vi "Set CPU Pools.vi"(8 "error in (no error)":errorcluster) -> (0 "error out":errorcluster, 2 "Processor Assignment":i32)   [LabVIEW 2014]
uses:
  <vilib>/Utility/RT CPU pool selections.ctl
  <vilib>/NI_Real-Time Target Support.lvlib
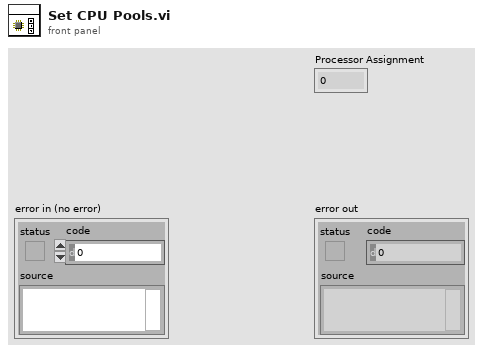
[diagram p1: front panel]
types:
  T1 = typedef "NI_Real-Time Target Support.lvlib/RT CPU pool selections.ctl" = enum16{"System & Timed Structures", "System", "Timed Structures", "Reserved"}
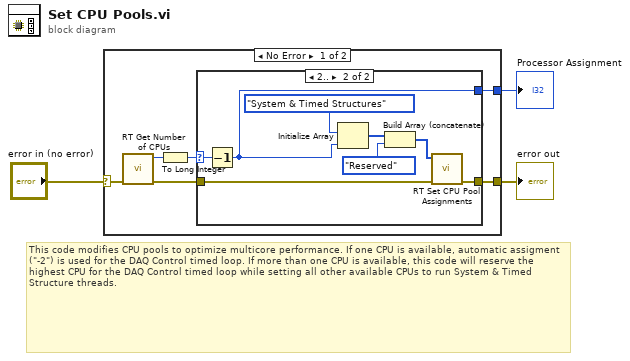
[diagram p0: block diagram]
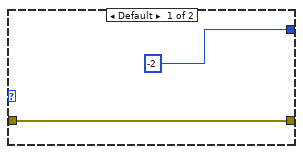
[diagram p2: hidden frame]
diagram:
  # "This code modifies CPU pools to optimize multicore performance. If one CPU is available, automatic assigment (\"-2\") is used for the DAQ Control timed loop. If more than one CPU is available, this code will reserve the highest CPU for the DAQ Control timed loop while setting all other available CPUs to run System & Timed Structure threads."
  n1 = case shown="No Error" "error in (no error)" {
    selector: "error in (no error)" -> [w7 w20]
    tunnel: [w8 w20] -> w3
    tunnel: [w5 _] -> w1
    frame No Error {
      n2 = call <vilib>:"RT Get Number of CPUs.vi"("error in (no error)"=w7) -> ("error out"=w9:errorcluster, "# of CPUs"=w6:u32)  [unwired: 9 in]
      n3 = To Long Integer(number=w6) -> (32bit integer=w4:i32)
      n4 = case shown="2.." w4 {
        selector: w4 -> [_ w13]
        tunnel: w9 -> [w11 w19]
        tunnel: [w11 w18] -> w8
        tunnel: [-2 ("# of CPUs") w12] -> w5
        frame Default {
        }
        frame 2.. {
          n5 = Decrement(x=w13) -> (x-1=w12:i32)
          n6 = Initialize Array(RT_CPU_pool_selections."System & Timed Structures" ("Enum"), w12) -> (w16:T1[])
          n7 = Build Array (concatenate)(w16, RT_CPU_pool_selections."Reserved" ("Enum")) -> (w14:T1[])
          n8 = call <vilib>:"RT Set CPU Pool Assignments.vi"("error in (no error)"=w19, "CPU pools"=w14) -> ("error out"=w18:errorcluster)  [unwired: 6 in, 3 out]
        }
      }
    }
    frame Error {
    }
  }
  "error out" <- w3
  "Processor Assignment" <- w1
